vi "Item_OnPopupMenu.vi"(11 "Object":T1) -> ()   [LabVIEW 2019, in "BlueSerializationProvider.lvlib"]
uses:
  BlueSerializationProvider.lvlib
  <resource>/Framework/Providers/API/ItemRef.ctl
  <resource>/Framework/Providers/API/mxLvMenuItem.ctl
panel:
  out "error out":errorcluster
  in  "error in":errorcluster
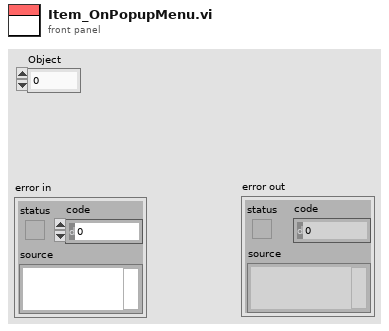
[diagram p1: front panel]
types:
  T1 = typedef "ItemRef.ctl" = u64
  T2 = typedef "mxLvMenuItem.ctl" = cluster{"Menu Name":string, "Description":string, "Icon File Name":path, "Menu Tag":string, "Enabled":bool, "Checked":bool, "Separator":bool, "Batchable":bool, "Weight":i32, "Batch Mode (Ignored if Not Batchable)":enum32{"Show If All Items Support Command", "Show If Any Items Support Command"}, "Menu Location":enum32{"<None>", "Project", "Project / Build Specifications", "Tools", "Tools / Source Control", "Tools / Real-Time Module", "Help"}, "Exclude From Getting Started Window Menu":bool}
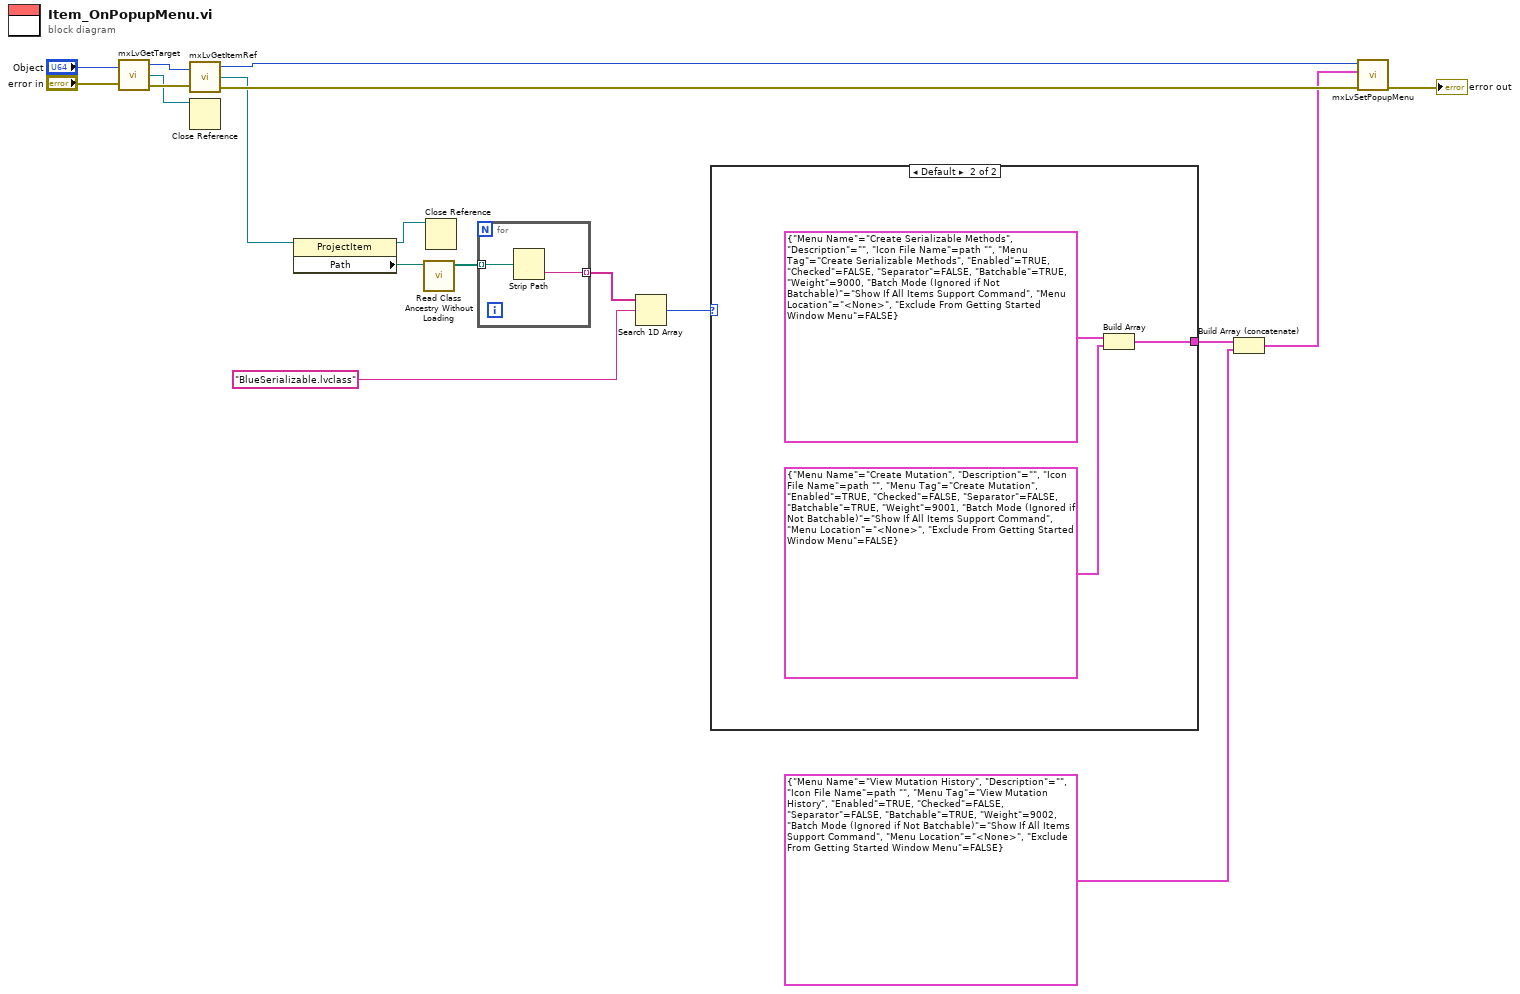
[diagram p0: block diagram]
diagram:
  n1 = call <resource>:"mxLvGetTarget.vi"("Item"="Object", "error in"="error in") -> ("Item"=w14:T1, "Target"=w11:refnum<vi>, "error out"=w12:errorcluster)
  n2 = call <resource>:"mxLvGetItemRef.vi"("Item"=w14, "error in"=w12) -> ("Item"=w17:T1, "Item Refnum"=w10:refnum<vi>, "error out"=w16:errorcluster)
  n3 = Close Reference(reference=w11) -> ()  [unwired: 1 in, 1 out]
  n4 = property class="ProjectItem"(reference=w10) -> (reference out=w5:refnum<vi>, "Path"=w9:path)  [unwired: 1 in, 1 out]
  n5 = call <vilib>:"Read Class Ancestry Without Loading.vi"("LabVIEW Class Path"=w9) -> ("Class Ancestry"=w8:path[])  [unwired: 9 in, 1 out]
  n6 = Close Reference(reference=w5) -> ()  [unwired: 1 in, 1 out]
  n7 = for {
    tunnel: w8 -> [w20] mode=indexing
    tunnel: [w19] -> w7 mode=indexing
    n8 = Strip Path(path=w20) -> (name=w19:string)  [unwired: 1 out]
  }
  n9 = Search 1D Array(1D array=w7, element="BlueSerializable.lvclass" ("name")) -> (index of element=w4:i32)  [unwired: 1 in]
  n10 = case shown="Default" w4 {
    tunnel: [_ w22] -> w3
    frame -1 {
    }
    frame Default {
      n11 = Build Array(T2 {"Menu Name"="Create Serializable Methods", "Description"="", "Icon File Name"=path "", "Menu Tag"="Create Serializable Methods", "Enabled"=TRUE, "Checked"=FALSE, "Separator"=FALSE, "Batchable"=TRUE, "Weight"=9000, "Batch Mode (Ignored if Not Batchable)"=enum."Show If All Items Support Command", "Menu Location"=enum."<None>", "Exclude From Getting Started Window Menu"=FALSE} ("Menu Item"), T2 {"Menu Name"="Create Mutation", "Description"="", "Icon File Name"=path "", "Menu Tag"="Create Mutation", "Enabled"=TRUE, "Checked"=FALSE, "Separator"=FALSE, "Batchable"=TRUE, "Weight"=9001, "Batch Mode (Ignored if Not Batchable)"=enum."Show If All Items Support Command", "Menu Location"=enum."<None>", "Exclude From Getting Started Window Menu"=FALSE} ("Menu Item")) -> (w22:T2[])
    }
  }
  n12 = Build Array (concatenate)(w3, T2 {"Menu Name"="View Mutation History", "Description"="", "Icon File Name"=path "", "Menu Tag"="View Mutation History", "Enabled"=TRUE, "Checked"=FALSE, "Separator"=FALSE, "Batchable"=TRUE, "Weight"=9002, "Batch Mode (Ignored if Not Batchable)"=enum."Show If All Items Support Command", "Menu Location"=enum."<None>", "Exclude From Getting Started Window Menu"=FALSE} ("Menu Item")) -> (w1:T2[])
  n13 = call <resource>:"mxLvSetPopupMenu.vi"("error in"=w16, "Popup Menu Items"=w1, "Item"=w17) -> ("error out"=→"error out":errorcluster)  [unwired: 7 in, 1 out]
